vi "testtt.vi"   [LabVIEW 2018]
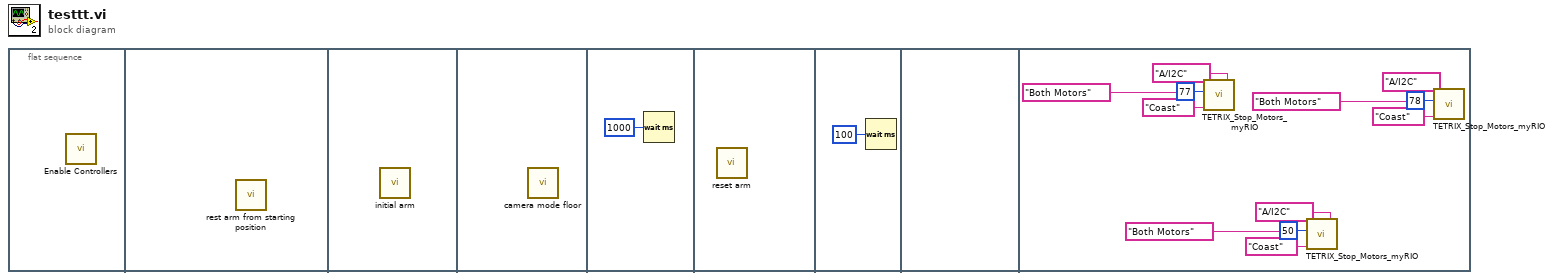
[diagram p0: block diagram]
diagram:
  n1 = flat-sequence {
    frame #0 {
      n2 = call "Enable Controllers.vi"() -> ()  [unwired: 12 in]
    }
    frame #1 {
      n3 = call "rest arm from starting position.vi"() -> ()  [unwired: 12 in]
    }
    frame #2 {
      n4 = call "initial arm.vi"() -> ()  [unwired: 12 in]
    }
    frame #3 {
      n5 = call "camera mode floor.vi"() -> ()  [unwired: 12 in]
    }
    frame #4 {
      n6 = Wait (ms)(milliseconds to wait=u32 1000) -> ()  [unwired: 1 out]
    }
    frame #5 {
      n7 = call "reset arm.vi"() -> ()  [unwired: 12 in]
    }
    frame #6 {
      n8 = Wait (ms)(milliseconds to wait=u32 100) -> ()  [unwired: 1 out]
    }
    frame #7 {
    }
    frame #8 {
      (unwired) tag "A/I2C" ("myRIO MXP Port A/B")
      n9 = call <vilib>:"TETRIX_Stop_Motors_myRIO.vi"("myRIO MXP Port A/B"=tag "A/I2C", "Stop Mode"="Coast", "Select Channel"="Both Motors", "Controller ID#  (I2C Address)"=u8 77) -> ()  [unwired: 3 in, 1 out]
      n10 = call <vilib>:"TETRIX_Stop_Motors_myRIO.vi"("myRIO MXP Port A/B"=tag "A/I2C", "Stop Mode"="Coast", "Select Channel"="Both Motors", "Controller ID#  (I2C Address)"=u8 50) -> ()  [unwired: 3 in, 1 out]
      n11 = call <vilib>:"TETRIX_Stop_Motors_myRIO.vi"("Stop Mode"="Coast", "Select Channel"="Both Motors", "Controller ID#  (I2C Address)"=u8 78) -> ()  [unwired: 4 in, 1 out]
    }
  }
